vi "Read REM IO VARs.vi"(7 "R/W Case":T7, 8 "error in (no error)":errorcluster, 9 "Output FIFO buffer in":dbl[](array[numeric]), 10 "I/O Output Data In":T1 {"BD Refs"."Data Reference" format="%.0x"}, 11 "I/O Output Vars in":T4[](array[typedef]) {"VS ref" format="%.0x"}) -> (0 "error out":errorcluster, 1 "Output FIFO buffer out":dbl[](array[numeric]), 2 "I/O Output Data Out":T1 {"BD Refs"."Data Reference" format="%.0x"}, 3 "I/O Output Vars out":T4[](array[typedef]) {"VS ref" format="%.0x"})   [LabVIEW 2019, in "SEECD Engine.lvlib"]
uses:
  SEECD Engine.lvlib
  Type Defs/RW Case.ctl
  Type Defs/REM IO ECAT Slave IOV Cluster.ctl
  <vilib>/NI VeriStand/Custom Device API/Custom Device Item Ref.ctl
  Type Defs/UDV Data Type.ctl
  Type Defs/Output Data.ctl
  <vilib>/NI VeriStand/Custom Device API/Block Data Reference.ctl
  <vilib>/NI VeriStand/Custom Device API/Data Reference.ctl
  <vilib>/NI VeriStand/Custom Device API/Global Data Refs.vi
  <vilib>/NI VeriStand/Custom Device API/Custom Device API.lvlib
  <vilib>/NI VeriStand/Custom Device Tools/Custom Device Utility Library/Custom Device Utility Library.lvlib
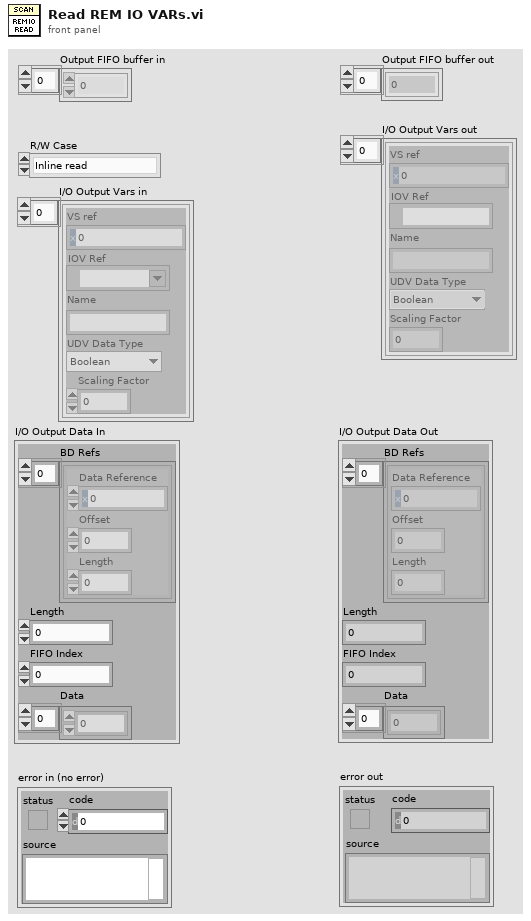
[diagram p1: front panel]
types:
  T1 = typedef "SEECD Engine.lvlib/Output Data.ctl" = cluster{"BD Refs":T2[], "Length":i32, "FIFO Index":i32, "Data":dbl[]}
  T2 = typedef "Custom Device API.lvlib/Block Data Reference.ctl" = cluster{"Data Reference":T3, "Offset":u64, "Length":u64}
  T3 = typedef "Custom Device API.lvlib/Data Reference.ctl" = i32
  T4 = typedef "SEECD Engine.lvlib/REM IO ECAT Slave IOV Cluster.ctl" = cluster{"VS ref":T5, "IOV Ref":refnum<k21>, "Name":string, "UDV Data Type":T6, "Scaling Factor":dbl}
  T5 = typedef "Custom Device API.lvlib/Custom Device Item Ref.ctl" = u64
  T6 = typedef "SEECD Engine.lvlib/UDV Data Type.ctl" = enum16{"Boolean", "Fixed Point", "Int8", "Int16", "Int32", "Int64", "U32 Bit Field", "UInt8", "UInt16", "UInt32", "UInt64", "Other", "DBL", "SGL"}
  T7 = typedef "SEECD Engine.lvlib/RW Case.ctl" = enum16{"Inline read", "Inline write", "Async - Inline loop read", "Async - Inline loop write", "Async loop (read/write)"}
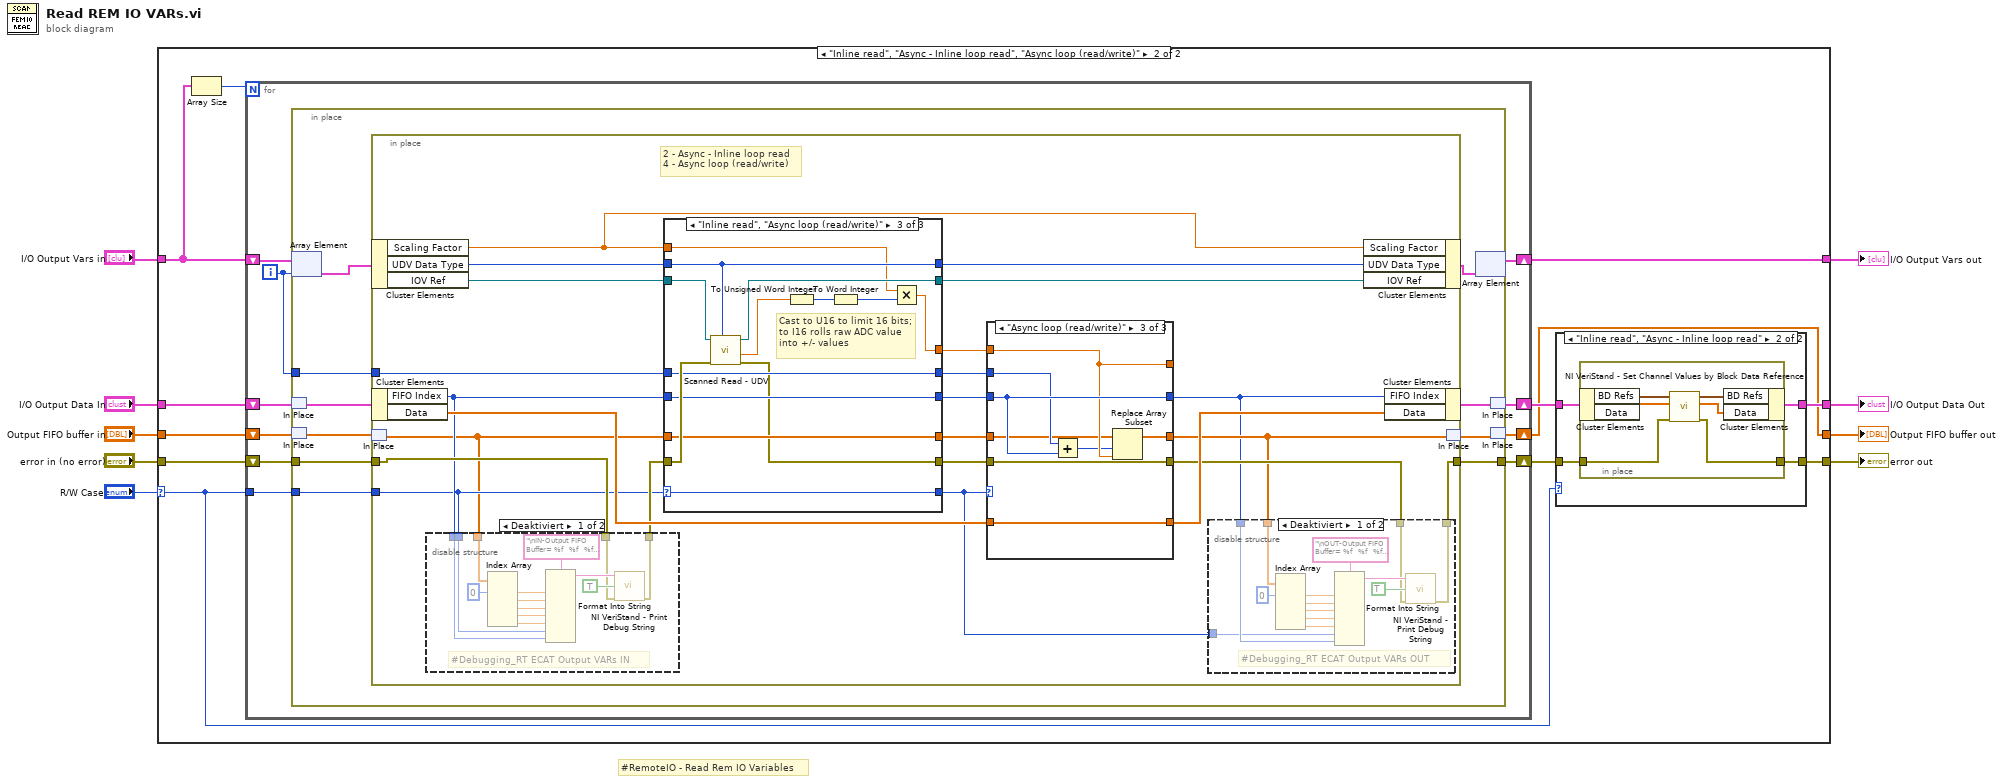
[diagram p0: block diagram]
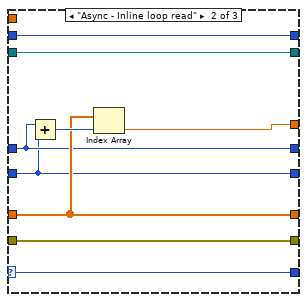
[diagram p4: hidden frame]
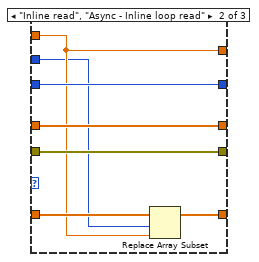
[diagram p6: hidden frame]
diagram:
  # "#RemoteIO - Read Rem IO Variables"
  n1 = case shown="\"Inline read\", \"Async - Inline loop read\", \"Async loop (read/write)\"" "R/W Case" {
    selector: "R/W Case" -> [_ w18]
    tunnel: [w11 w14] -> w9
    tunnel: "Output FIFO buffer in" -> [w11 w25]
    tunnel: [w12 w15] -> w1
    tunnel: [w13 w24] -> w3
    tunnel: "I/O Output Data In" -> [w12 w23]
    tunnel: "I/O Output Vars in" -> [w13 w22]
    tunnel: [w10 w16] -> w7
    tunnel: "error in (no error)" -> [w10 w20]
    frame Default {
    }
    frame "Inline read", "Async - Inline loop read", "Async loop (read/write)" {
      n2 = Array Size(array=w22) -> (size(s)=w21:i32)
      n3 = for {
        N: w21 -> [_]
        shift-right: [w34] -> w24
        shift-left: w22 -> [w35]
        shift-right: [w26] -> w19
        shift-left: w23 -> [w29]
        shift-right: [w32] -> w14
        shift-left: w25 -> [w33]
        shift-right: [w30] -> w17
        shift-left: w20 -> [w31]
        tunnel: w18 -> [w28]
        i -> [w27]
        n4 = in-place {
          in-place-border: w31 -> [w43]
          in-place-border: [w37] -> w30
          in-place-border: w28 -> [w42]
          in-place-border: w27 -> [w41]
          n5 = in-place-array #1(w35, w27) -> (w36:T4)
          n6 = in-place-match #2(w29) -> (w45:T1)
          n7 = in-place-match #3(w33) -> (w44:dbl[])
          n8 = in-place {
            in-place-border: w43 -> [w59]
            in-place-border: w42 -> [w56]
            in-place-border: w41 -> [w65]
            in-place-border: [w53] -> w37
            # "2 - Async - Inline loop read\n4 - Async loop (read/write)"
            n9 = in-place-cluster #4(w36) -> ("Scaling Factor"=w46:dbl, "UDV Data Type"=w67:T6, "IOV Ref"=w66:refnum<k21>)
            n10 = in-place-cluster #5(w45) -> ("FIFO Index"=w57:i32, "Data"=w68:dbl[])
            n11 = in-place-match #6(w44) -> (w55:dbl[])
            n12 = disable-structure shown="Deaktiviert" {
              disable-tunnel: w59 -> [w138 w148]
              disable-tunnel: [w137 w148] -> w58
              disable-tunnel: w57 -> [w136 _]
              disable-tunnel: w56 -> [w135 _]
              disable-tunnel: w55 -> [w134 _]
              frame Disabled {
                # "#Debugging_RT ECAT Output VARs IN"
                n13 = Index Array(array=w134, index #1=0) -> (element #1=w142:dbl, element #2=w141:dbl, element #3=w140:dbl, element #4=w139:dbl, element #5=w147:dbl)  [unwired: 4 in]
                n14 = Format Into String(format string="\nIN-Output FIFO Buffer= %f   %f   %f   %f   %f   - MODE: %d  - Index: %d\n" ("Format-String"), w142, w141, w140, w139, w147, w135, w136) -> (resulting string=w145:string)  [unwired: 2 in, 1 out]
                n15 = call <vilib>:"NI VeriStand - Print Debug String.vi"("error in (no error)"=w138, "Add to log file? (F)"=TRUE, "Message"=w145) -> ("error out"=w137:errorcluster)  [unwired: 8 in]
              }
              frame Enabled {
              }
            }
            n16 = case shown="\"Inline read\", \"Async loop (read/write)\"" w56 {
              selector: w56 -> [w69 w79 w90]
              tunnel: w67 -> [w70 w77 w91]
              tunnel: w66 -> [w71 w78 w98]
              tunnel: w57 -> [w73 w80 w94]
              tunnel: w55 -> [w74 w83 w93]
              tunnel: [w74 w83 w93] -> w61
              tunnel: w65 -> [w72 w81 w95]
              tunnel: [_ w82 w89] -> w49
              tunnel: [w72 w81 w95] -> w63
              tunnel: [w73 w80 w94] -> w62
              tunnel: [w69 w79 w90] -> w50
              tunnel: [w71 w78 w97] -> w47
              tunnel: [w70 w77 w91] -> w64
              tunnel: w58 -> [w75 w76 w96]
              tunnel: [w75 w76 w92] -> w48
              tunnel: w46 -> [_ _ w85]
              frame Default {
              }
              frame "Async - Inline loop read" {
                n17 = Add(x=w81, y=w80) -> (x+y=w84:i32)
                n18 = Index Array(array=w83, index=w84) -> (element=w82:dbl)
              }
              frame "Inline read", "Async loop (read/write)" {
                # "Cast to U16 to limit 16 bits;\nto I16 rolls raw ADC value\ninto +/- values"
                n19 = call "Scanned Read - UDV.vi"("UDV Data Type"=w91, "error in (no error)"=w96, "IOV ref in"=w98) -> ("error out"=w92:errorcluster, "data out"=w88:dbl, "IOV ref out"=w97:refnum<k21>)  [unwired: 6 in]
                n20 = To Unsigned Word Integer(number=w88) -> (unsigned 16bit integer=w86:u16)
                n21 = To Word Integer(number=w86) -> (16bit integer=w87:i16)
                n22 = Multiply(x=w85, y=w87) -> (x*y=w89:dbl)
              }
            }
            n23 = case shown="\"Async loop (read/write)\"" w50 {
              tunnel: w63 -> [_ w104 w114]
              tunnel: w62 -> [w99 w106 w115]
              tunnel: w49 -> [w100 w105 w113]
              tunnel: w61 -> [w101 w107 w112]
              tunnel: w48 -> [w102 w108 w117]
              tunnel: w68 -> [w103 w110 w116]
              tunnel: [w99 w106 w115] -> w51
              tunnel: [w103 w109 w116] -> w60
              tunnel: [w102 w108 w117] -> w54
              tunnel: [w101 w107 w118] -> w52
              tunnel: [w100 w105 w113] -> _
              frame Default {
              }
              frame "Inline read", "Async - Inline loop read" {
                n24 = Replace Array Subset(array=w110, new element=w105, index=w104) -> (w109:dbl[])
              }
              frame "Async loop (read/write)" {
                n25 = Add(x=w114, y=w115) -> (x+y=w111:i32)
                n26 = Replace Array Subset(array=w112, new element=w113, index=w111) -> (w118:dbl[])
              }
            }
            n27 = disable-structure shown="Deaktiviert" {
              disable-tunnel: w54 -> [w123 w133]
              disable-tunnel: [w122 w133] -> w53
              disable-tunnel: w52 -> [w121 _]
              disable-tunnel: w51 -> [w120 _]
              disable-tunnel: w50 -> [w119 _]
              frame Disabled {
                # "#Debugging_RT ECAT Output VARs OUT"
                n28 = Index Array(array=w121, index #1=0) -> (element #1=w127:dbl, element #2=w126:dbl, element #3=w125:dbl, element #4=w124:dbl, element #5=w132:dbl)  [unwired: 4 in]
                n29 = Format Into String(format string="\nOUT-Output FIFO Buffer= %f   %f   %f   %f   %f   - MODE: %d  - Index: %d\n" ("Format-String"), w127, w126, w125, w124, w132, w119, w120) -> (resulting string=w130:string)  [unwired: 2 in, 1 out]
                n30 = call <vilib>:"NI VeriStand - Print Debug String.vi"("error in (no error)"=w123, "Add to log file? (F)"=TRUE, "Message"=w130) -> ("error out"=w122:errorcluster)  [unwired: 8 in]
              }
              frame Enabled {
              }
            }
            n31 = in-place-cluster #4("Scaling Factor"=w46, "UDV Data Type"=w64, "IOV Ref"=w47) -> (w40:T4)
            n32 = in-place-cluster #5("FIFO Index"=w51, "Data"=w60) -> (w39:T1)
            n33 = in-place-match #6(w52) -> (w38:dbl[])
          }
          n34 = in-place-array #1(w40) -> (w34:T4[])  [unwired: 1 out]
          n35 = in-place-match #2(w39) -> (w26:T1)
          n36 = in-place-match #3(w38) -> (w32:dbl[])
        }
      }
      n37 = case shown="\"Inline read\", \"Async - Inline loop read\"" w18 {
        tunnel: w19 -> [w149 w151]
        tunnel: w17 -> [w150 w154]
        tunnel: [w150 w153] -> w16
        tunnel: [w149 w152] -> w15
        frame Default {
        }
        frame "Inline read", "Async - Inline loop read" {
          n38 = in-place {
            in-place-border: w154 -> [w158]
            in-place-border: [w157] -> w153
            n39 = in-place-cluster #7(w151) -> ("BD Refs"=w156:T2[], "Data"=w155:dbl[])
            n40 = call <vilib>:"NI VeriStand - Set Channel Values by Block Data Reference.vi"("error in (no error)"=w158, "Values Array in"=w155, "Block Data Ref"=w156) -> ("error out"=w157:errorcluster, "Values Array out"=w159:dbl[], "Block Data Ref dup"=w160:T2[])  [unwired: 6 in]
            n41 = in-place-cluster #7("BD Refs"=w160, "Data"=w159) -> (w152:T1)
          }
        }
      }
    }
  }
  "Output FIFO buffer out" <- w9
  "error out" <- w7
  "I/O Output Vars out" <- w3
  "I/O Output Data Out" <- w1
